vi "SCVac_readback.vi"(11 "Readback array":string[](array[string])) -> (1 "6600 V1":dbl, 2 "Scatt TC (Torr)":string, 3 "Scat. Chamber":string, 4 "6600 V3":dbl)   [LabVIEW 2014]
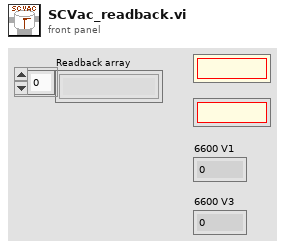
[diagram p1: front panel]
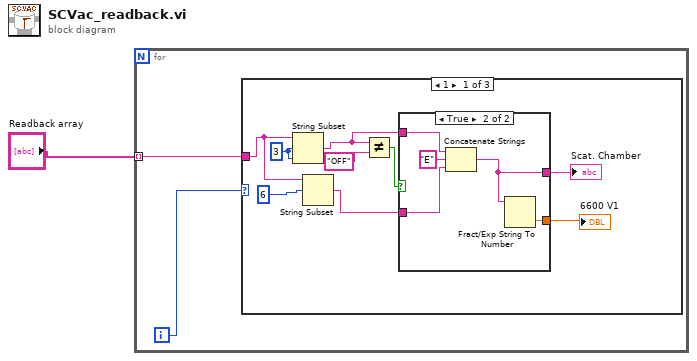
[diagram p0: block diagram]
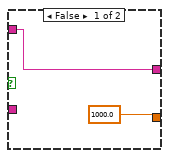
[diagram p2: hidden frame]
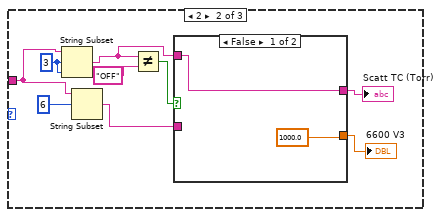
[diagram p3: hidden frame]
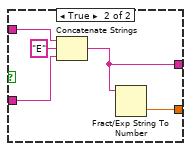
[diagram p4: hidden frame]
diagram:
  n1 = for {
    tunnel: "Readback array" -> [w2] mode=indexing
    i -> [w3]
    n2 = case shown="1" w3 {
      tunnel: w2 -> [w9 w25 _]
      frame 1 {
        w11 = 3 ("offset (0)")
        n3 = String Subset(string=w9, offset (0)=w11, length (rest)=w11) -> (substring=w6:string)
        n4 = String Subset(string=w9, offset (0)=6 ("length (rest)")) -> (substring=w8:string)  [unwired: 1 in]
        n5 = Not Equal?(x=w6, y="OFF") -> (x != y?=w7:bool)
        n6 = case shown="True" w7 {
          tunnel: w8 -> [_ w17]
          tunnel: w6 -> [w14 w18]
          tunnel: [w14 w16] -> w5
          tunnel: [1000.0 w15] -> w4
          frame False {
          }
          frame True {
            n7 = Concatenate Strings(w18, "E" ("string"), w17) -> (w16:string)
            n8 = Fract/Exp String To Number(string=w16) -> (number=w15:dbl)  [unwired: 3 in, 1 out]
          }
        }
        "Scat. Chamber" <- w5
        "6600 V1" <- w4
      }
      frame 2 {
        w27 = 3 ("offset (0)")
        n9 = String Subset(string=w25, offset (0)=w27, length (rest)=w27) -> (substring=w22:string)
        n10 = String Subset(string=w25, offset (0)=6 ("length (rest)")) -> (substring=w24:string)  [unwired: 1 in]
        n11 = Not Equal?(x=w22, y="OFF") -> (x != y?=w23:bool)
        n12 = case shown="False" w23 {
          tunnel: w24 -> [_ w33]
          tunnel: w22 -> [w30 w34]
          tunnel: [w30 w32] -> w20
          tunnel: [1000.0 w31] -> w21
          frame False {
          }
          frame True {
            n13 = Concatenate Strings(w34, "E" ("string"), w33) -> (w32:string)
            n14 = Fract/Exp String To Number(string=w32) -> (number=w31:dbl)  [unwired: 3 in, 1 out]
          }
        }
        "6600 V3" <- w21
        "Scatt TC (Torr)" <- w20
      }
      frame 0, Default {
      }
    }
  }
